vi "AlliGator Create Individual Pixel ROIs from ROI.vi"(5 "Y Resolution":i32, 7 "X Resolution":i32, 8 "Error In":errorcluster, 9 "Abort ROI Creation":refnum<vi>, 10 "Selected ROI (-1: use ROI Descriptor)":i32=-1, 11 "ROI":T1 {"Contours"."Type" items=["No Selection", "Point", "Line", "Rectangle", "Oval", "Polygon", "Freehand Region", "Annulus", "Unused2", "Unused3", "Broken Line", "Freehand Line", "Rotated Rectangle"]}) -> (0 "Error Out":errorcluster, 2 "Message":string)   [LabVIEW 2021, in "AlliGator ROIs.lvlib"]
doc: "Converts a closed ROI into a series of single-pixel ROIs."
uses:
  AlliGator ROIs.lvlib
  AlliGator Variables List.ctl
  AlliGator ROI Manager Actions.ctl
  Image/Named ROI Description.ctl
  Variant/Variant to Data/Variant to I32.vi
  AlliGator Source Image ROI Storage [SGL] v3.vi
  AlliGator Source Image ROI Storage [MULT] v3.vi
  AlliGator Globals, Variables & Constants.lvlib
  Variant/Variant to Data/Variant to Data.lvlib
  Image/Image.lvlib
  Error/Error.lvlib
  Utilities/Utilities.lvlib
panel:
  # "see the AlliGator License on the block diagram (Ctrl+E or Window:Show Block Diagram)"
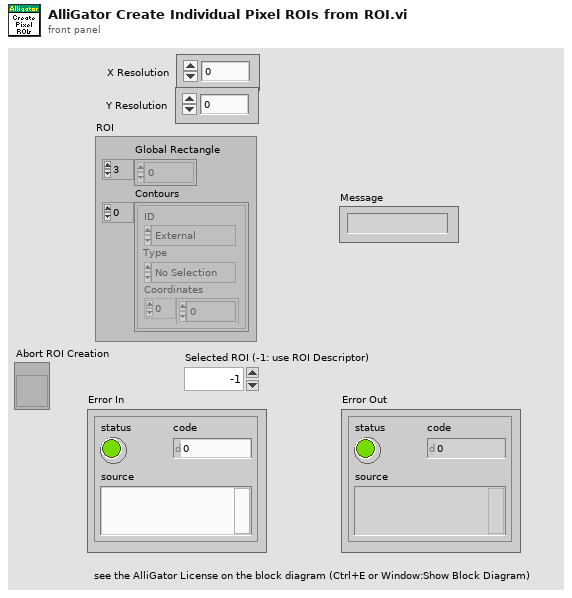
[diagram p1: front panel]
types:
  T1 = typedef "ROI Descriptor" = cluster{"Global Rectangle":i32[], "Contours":cluster{"ID":enum32{"External", "Internal"}, "Type":u32, "Coordinates":i32[]}[]}
  T2 = typedef "AlliGator Globals, Variables & Constants.lvlib/AlliGator Variables List.ctl" = enum16{"---- GUI ----", "GUI:Initialization Status", "GUI:State Indicators Refnum", "GUI:Original AlliGator Menu Items", "GUI:Current Action Loop State", "GUI:Script in progress", "GUI:Playback", "GUI:Loop Playback", "GUI:Search ROI Used", "GUI:Search ROI", "Decay Graph Max Legend Size", "Intensity Graph Max Legend Size", "Decay Statistics Graph Max Legend Size", "Phasor Graph Max Legend Size", "Phasor Ratio Graph Max Legend Size", "Lifetime Graph Max Legend Size", "---- Files ----", "Files:Export Dataset Frames as Individual Files", "Files:Show Batch Export Help Balloons", "Files:Frames in Dataset", "Files:ptu File Frame Start Indices", "Files:Current Frame in Dataset", "Files:Current Frame Timestamp", "Files:Dataset Loaded", "Files:Dataset Metadata", "Files:Dataset Channel", "Files:Dataset Data Description", "Files:Background Dataset Metadata", "Files:Background Dataset Channel", "Files:Background Dataset Data Description", "Files:Background File Subtraction", "Files:Background File Path", "Files:Background File Pile-up Correction", "Files:Background File Pixel Well Capacity", "Files:Background File Scaling Factor", "Files:Current Dataset Load Settings", "Files:Dataset Path", "Files:ICCD-specific Information", "Files:Macrotime Gate Separation", "------ Python Plugins ------", "Python Plugins:Information", "Python Plugins:Python Session", "Python Plugins:Valid Python Session?", "---- Source Image ----", "Source Image:ROIs", "Source Image:Current ROI", "Source Image:ROI Event Refnum", "X_Source Image Display Range", "X_Source Image Palette Information", "X_Type of Displayed Image", "X_Time Gate Slider", "Source Image:Palette List", "Source Image:Scale", "Source Image:ROI Overlay Color", "Source Image:Overlay to Erase", "Source Image:Is Displayed Image Accumulated", "Source Image:White Light Image Modified", "Source Image:Mask Image Modified", "---- Image Profile Window ----", "Image Profile:Window Event Refnum", "Image Profile:IntensityType", "Image Profile:Intensity Average Type", "Image Profile:Intensity-weighted SDV", "Image Profile:Box Profile Type", "Image Profile:Window Open", "Image Profile:Plotted Fit Parameter", "------ Phasor Graph -------", "Phasor Graph:Show Line", "---- Phasor Plot ---", "Phasor Plot:Parameters Changed", "Phasor Plot:FLI Dataset Modified since last Calculation", "Phasor Harmonics Data", "Selected Phasor Harmonics", "Phasor Harmonic Manager Event Refnum", "Phasor Plot:ROIs", "Phasor Plot:Current ROI", "Phasor Plot:ROI Event Refnum", "Phasor Plot:Image Reference Points", "Phasor Plot:Computed", "Phasor Plot:Palette Information", "Phasor Plot:Palette List", "Phasor Plot:Phasor Ratio Palette Information", "Phasor Plot:Phasor Ratio Palette List", "Phasor Plot:Image Scale", "Phasor Plot:Image Overlay to Erase", "Phasor Plot:Image Elements to Update", "Phasor Plot:Current Calculation Parameters", "Phasor Plot:Current Calibration Options", "Phasor Plot:Reset Cumulated Phasor Plot", "Phasor Plot:Reference 1", "Phasor Plot:Lifetime Reference 1", "Phasor Plot:Reference 1 Frequency", "Phasor Plot:Reference 2", "Phasor Plot:Lifetime Reference 2", "Phasor Plot:Reference 2 Frequency", "---- Decay Analysis ----", "Number of Selected Decays to Fit", "LS Fit Results", "LAR Fit Results", "BS Fit Results", "Last Decay Max - Min", "Best Fit Parameters", "Best Fit Parameter Names", "Actual Size X", "Actual Size Y", "Binning X", "Binning Y", "Actual # Gates", "Dataset Number", "Gates to...", "Gates Skipped", "Gates to keep", "Gate Step", "Gate Separation", "Reversed Gates", "Pile-up Correction", "Pixel Well Capacity", "Background Subtracted", "Background Subtraction Method", "Background Definition Range", "Background File (deprecated)", "Number of Dataset Accumulated", "Array of Accumulated Dataset Paths", "Do Averaged Datasets", "Destination File Path", "Process Plot Target", "Use 1/D as Phasor Frequency", "---- Decay Fit Parameter Map -----", "Decay Fit Parameter Map:Palette Information", "Decay Fit Parameter Map:Palette List", "------- Local Decay Window ---------", "Local Decay Graph Window:Event Refnum", "Local Decay Graph Window:Use normalized IRF for convolution", "----- Miscellaneous ----", "Misc:Skippable Dialog Windows Status"}
  T3 = typedef "AlliGator ROIs.lvlib/AlliGator ROI Manager Actions.ctl" = enum16{"Undefined", "Delete Current ROI", "Delete All Unselected ROIs", "Delete Multiple ROIs", "Delete All ROIs", "Swap ROIs", "Insert ROI", "Update Current ROI Descriptor", "Rename Current ROI", "Store New ROI", "Store Multiple ROIs", "Select Next ROI", "Select Previous ROI", "Find Selected ROI", "Show All ROIs", "Update ROI Manager Window", "Merge All ROIs", "Unmerge ROI", "Set Selected ROI by ID"}
  T4 = typedef "Image.lvlib/Named ROI Description.ctl" = cluster{"ROI Descriptor":T1, "ROI Name":string, "Overlay Color":u32}
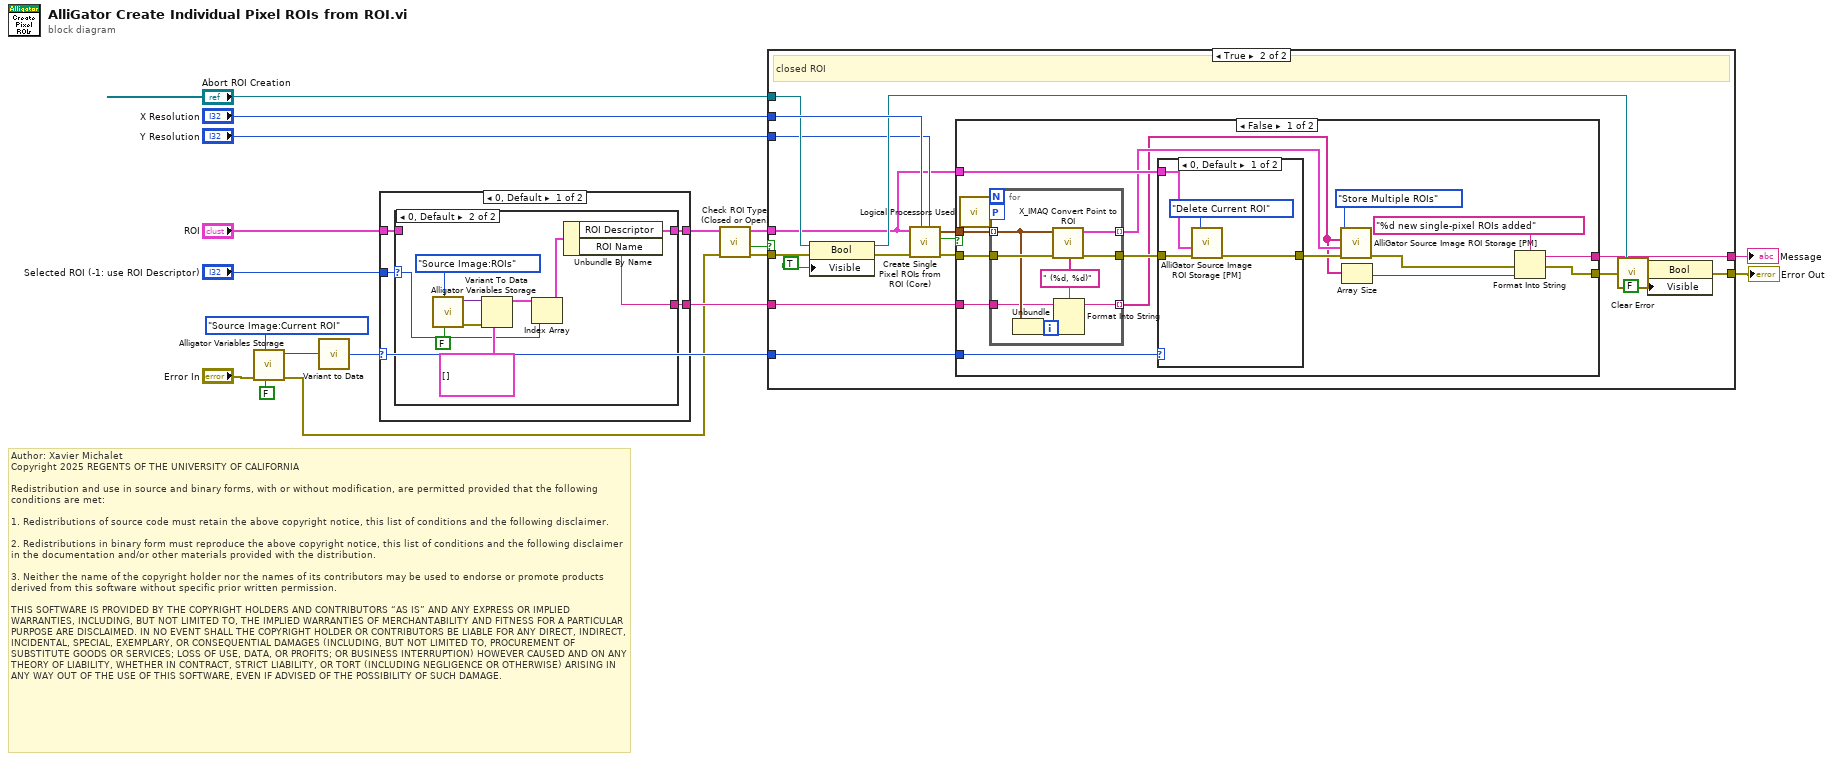
[diagram p0: block diagram]
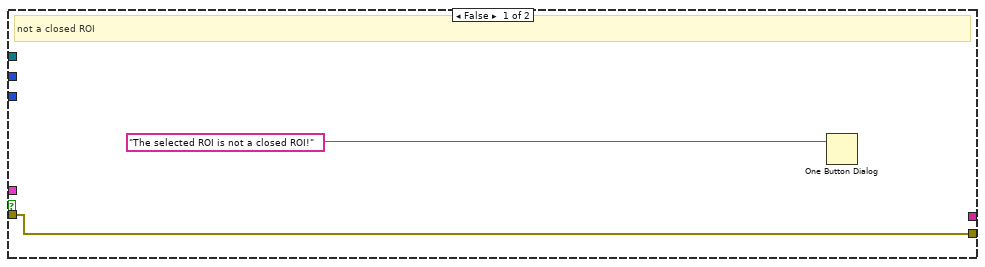
[diagram p2: hidden frame]
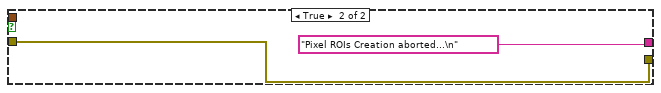
[diagram p4: hidden frame]
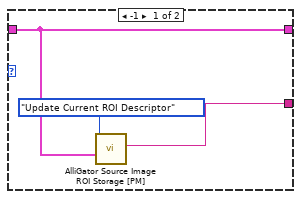
[diagram p5: hidden frame]
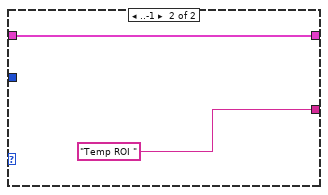
[diagram p6: hidden frame]
diagram:
  # "Author: Xavier Michalet\nCopyright 2025 REGENTS OF THE UNIVERSITY OF CALIFORNIA\n\nRedistribution and use in source and binary forms, with or without modification, are permitted provided that the following conditions are met:\n\n1. Redistributions of source code must retain the above copyright notice, this list of conditions and the following disclaimer.\n\n2. Redistributions in binary form must reproduce the above copyright notice, this list of conditions and the following disclaimer in the documentation and/or other materials provided with the distribution.\n\n3. Neither the name of the copyright holder nor the names of its contributors may be used to endorse or promote products derived from this software without specific prior written permission.\n\nTHIS SOFTWARE IS PROVIDED BY THE COPYRIGHT HOLDERS AND CONTRIBUTORS “AS IS” AND ANY EXPRESS OR IMPLIED WARRANTIES, INCLUDING, BUT NOT LIMITED TO, THE IMPLIED WARRANTIES OF MERCHANTABILITY AND FITNESS FOR A PARTICULAR PURPOSE ARE DISCLAIMED. IN NO EVENT SHALL THE COPYRIGHT HOLDER OR CONTRIBUTORS BE LIABLE FOR ANY DIRECT, INDIRECT, INCIDENTAL, SPECIAL, EXEMPLARY, OR CONSEQUENTIAL DAMAGES (INCLUDING, BUT NOT LIMITED TO, PROCUREMENT OF SUBSTITUTE GOODS OR SERVICES; LOSS OF USE, DATA, OR PROFITS; OR BUSINESS INTERRUPTION) HOWEVER CAUSED AND ON ANY THEORY OF LIABILITY, WHETHER IN CONTRACT, STRICT LIABILITY, OR TORT (INCLUDING NEGLIGENCE OR OTHERWISE) ARISING IN ANY WAY OUT OF THE USE OF THIS SOFTWARE, EVEN IF ADVISED OF THE POSSIBILITY OF SUCH DAMAGE."
  n1 = call "Alligator Variables Storage.vi"("Get(F)/Set"=FALSE, "AlliGator Variable"=AlliGator_Variables_List."Source Image:Current ROI" ("Alligator Variable"), "Error In"="Error In") -> ("Error Out"=w4:errorcluster, "Data out"=w16:variant)  [unwired: 6 in, 1 out]
  n2 = call-poly "Variant to Data.vi"("Variant"=w16) -> ("Value"=w12:i32)  [unwired: 8 in]
  n3 = case shown="0, Default" w12 {
    tunnel: [w21 "Temp ROI " ("Current ROI Name")] -> w15
    tunnel: "ROI" -> [w22 w36]
    tunnel: [w20 w36] -> w6
    tunnel: "Selected ROI (-1: use ROI Descriptor)" -> [w19 _]
    frame 0, Default {
      n4 = case shown="0, Default" w19 {
        selector: w19 -> [_ w26]
        tunnel: w22 -> [w23 _]
        tunnel: [w25 w27] -> w21
        tunnel: [w23 w28] -> w20
        frame -1 {
          n5 = call-poly "AlliGator Source Image ROI Storage [PM].vi"("Current ROI Descriptor"=w23, "Action"=AlliGator_ROI_Manager_Actions."Update Current ROI Descriptor" ("Enum")) -> ("Current ROI Name"=w25:string)  [unwired: 3 in, 6 out]
        }
        frame 0, Default {
          n6 = call "Alligator Variables Storage.vi"("Get(F)/Set"=FALSE, "AlliGator Variable"=AlliGator_Variables_List."Source Image:ROIs" ("Alligator Variable")) -> ("Error Out"=w33:errorcluster, "Data out"=w34:variant)  [unwired: 7 in, 1 out]
          n7 = Variant To Data(error in=w33, type=T4[] [] ("Stored ROIs in"), Variant=w34) -> (data=w30:T4[])  [unwired: 1 out]
          n8 = Index Array(array=w30, index=w26) -> (element=w29:T4)
          n9 = Unbundle By Name(w29) -> ("ROI Descriptor"=w28:T1, "ROI Name"=w27:string)
        }
      }
    }
    frame ..-1 {
    }
  }
  n10 = call "Check ROI Type (Closed or Open).vi"("Error In"=w4, "ROI Descriptor"=w6) -> ("Error Out"=w3:errorcluster, "Closed ROI"=w1:bool, "ROI Descriptor dup"=w5:T1)  [unwired: 5 in, 2 out]
  n11 = case shown="True" w1 {
    tunnel: w15 -> [_ w43]
    tunnel: "X Resolution" -> [_ w57]
    tunnel: "Y Resolution" -> [_ w49]
    tunnel: w12 -> [_ w44]
    tunnel: [_ w41] -> w9
    tunnel: [w39 w40] -> w8
    tunnel: w5 -> [_ w45]
    tunnel: w3 -> [w39 w51]
    tunnel: "Abort ROI Creation" -> [_ w53]
    frame False {
      # "not a closed ROI"
      n12 = One Button Dialog(message="The selected ROI is not a closed ROI!") -> ()  [unwired: 1 in, 1 out]
    }
    frame True {
      # "closed ROI"
      n13 = property class="Bool"(reference=w53, error in=w51, "Visible"=TRUE) -> (reference out=w52:refnum<vi>, error out=w50:errorcluster)
      n14 = call "Create Single Pixel ROIs from ROI (Core).vi"("Y Resolution"=w49, "X Resolution"=w57, "error in (no error)"=w50, "ROI Descriptor"=w45) -> ("error out"=w46:errorcluster, "Aborted"=w47:bool, "Point Array"=w48:cluster{"Numeric":i32, "Numeric":i32}[])  [unwired: 5 in]
      n15 = case shown="False" w47 {
        tunnel: [w58 w89] -> w42
        tunnel: [w71 "Pixel ROIs Creation aborted...\n" ("Prefix (\"\")")] -> w41
        tunnel: w48 -> [w64 _]
        tunnel: w46 -> [w66 w89]
        tunnel: w44 -> [w68 _]
        tunnel: w45 -> [w67 _]
        tunnel: w43 -> [w62 _]
        frame False {
          n16 = call "Logical Processors Used.vi"() -> ("# Logical Processor Used"=w63:i32)  [unwired: 6 in]
          n17 = for {
            tunnel: w66 -> [w82]
            tunnel: [w81] -> w65
            tunnel: w64 -> [w78] mode=indexing
            tunnel: [w80] -> w61 mode=indexing
            workers-P: w63 -> [_]
            tunnel: w62 -> [w75]
            tunnel: [w74] -> w60 mode=indexing
            n18 = Unbundle(w78) -> ("Numeric"=w77:i32, "Numeric"=w76:i32)
            n19 = call "X_IMAQ Convert Point to ROI.vi"("error in (no error)"=w82, "Point"=w78) -> ("error out"=w81:errorcluster, "ROI Descriptor"=w80:T1)  [unwired: 7 in]
            n20 = Format Into String(format string=" (%d, %d)", initial string=w75, w77, w76) -> (resulting string=w74:string)  [unwired: 1 in, 1 out]
          }
          n21 = case shown="0, Default" w68 {
            tunnel: w65 -> [w85 w87]
            tunnel: [w84 w87] -> w69
            tunnel: w67 -> [w83 _]
            frame 0, Default {
              n22 = call-poly "AlliGator Source Image ROI Storage [PM].vi"("Error In"=w85, "Current ROI Descriptor"=w83, "Action"=AlliGator_ROI_Manager_Actions."Delete Current ROI") -> ("Error Out"=w84:errorcluster)  [unwired: 2 in, 6 out]
            }
            frame ..-1 {
            }
          }
          n23 = call-poly "AlliGator Source Image ROI Storage [PM].vi"("Error In"=w69, "Current ROI Descriptors"=w61, "Default Names (\"ROI\")"=w60, "Action"=AlliGator_ROI_Manager_Actions."Store Multiple ROIs") -> ("Error Out"=w59:errorcluster)  [unwired: 2 in, 5 out]
          n24 = Array Size(array=w60) -> (size(s)=w73:i32)
          n25 = Format Into String(format string="%d new single-pixel ROIs added" ("Prefix (\"\")"), error in=w59, w73) -> (resulting string=w71:string, error out=w58:errorcluster)  [unwired: 1 in]
        }
        frame True {
        }
      }
      n26 = call "Clear Error.vi"("Error In"=w42) -> ("no Error Out"=w56:errorcluster)  [unwired: 8 in]
      n27 = property class="Bool"(reference=w52, error in=w56, "Visible"=FALSE) -> (error out=w40:errorcluster)  [unwired: 1 out]
    }
  }
  "Error Out" <- w8
  "Message" <- w9
